vi "AB_RW_Project_Source_VI.vi"(7 "action":T3, 8 "error in (no error)":errorcluster, 9 "index in":i32, 10 "dataSource in":T2, 11 "buildObject":T1) -> (0 "error out":errorcluster, 1 "index out":i32, 2 "dataSource out":T2, 3 "buildObject out":T1)   [LabVIEW 2020]
doc: "Reads and writes the data to the object property bag."
uses:
  <resource>/Framework/Providers/API/ItemRef.ctl
  <vilib>/AppBuilder/RW_Project/AB_RW_Project_Source_VI_Data.ctl
  <vilib>/AppBuilder/RW_Project/AB_RW_Project_PropBag_Action.ctl
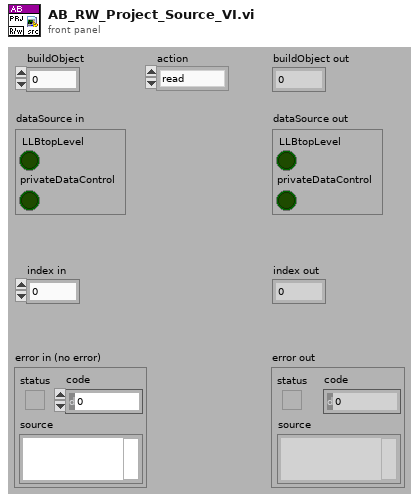
[diagram p1: front panel]
types:
  T1 = typedef "ItemRef.ctl" = u64
  T2 = typedef "AB_RW_Project_Source_VI_Data.ctl" = cluster{"LLBtopLevel":bool, "privateDataControl":bool}
  T3 = typedef "AB_RW_Project_PropBag_Action.ctl" = enum16{"read", "write", "clear", "readPrevious", "writePrevious", "clearPrevious"}
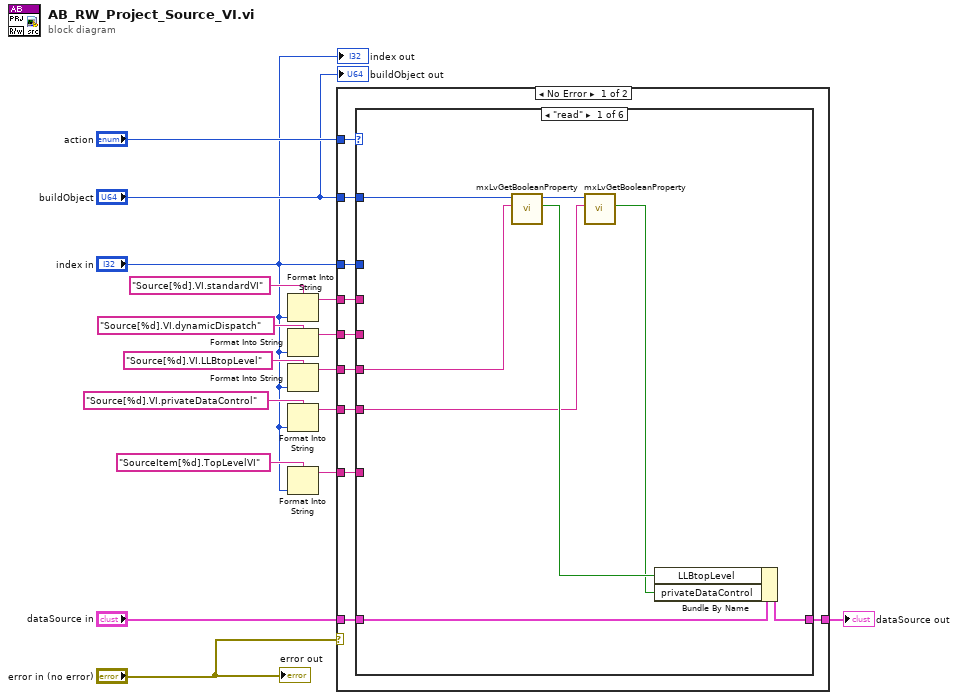
[diagram p0: block diagram]
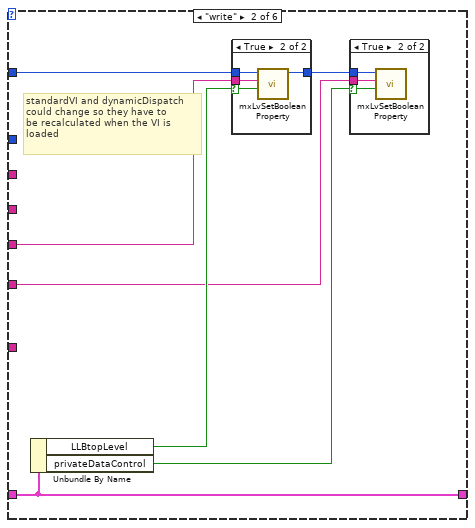
[diagram p2: hidden frame]
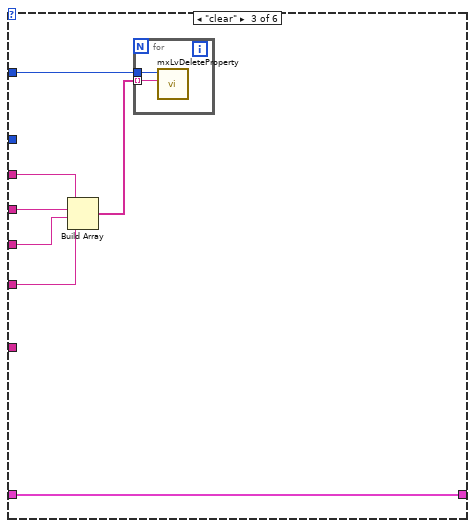
[diagram p5: hidden frame]
diagram:
  n1 = Format Into String(format string="Source[%d].VI.standardVI", "index in") -> (resulting string=w13:string)  [unwired: 2 in, 1 out]
  n2 = Format Into String(format string="Source[%d].VI.dynamicDispatch", "index in") -> (resulting string=w10:string)  [unwired: 2 in, 1 out]
  n3 = Format Into String(format string="Source[%d].VI.LLBtopLevel", "index in") -> (resulting string=w9:string)  [unwired: 2 in, 1 out]
  n4 = Format Into String(format string="Source[%d].VI.privateDataControl", "index in") -> (resulting string=w1:string)  [unwired: 2 in, 1 out]
  n5 = Format Into String(format string="SourceItem[%d].TopLevelVI", "index in") -> (resulting string=w4:string)  [unwired: 2 in, 1 out]
  n6 = case shown="No Error" "error in (no error)" {
    tunnel: "action" -> [w26 _]
    tunnel: "dataSource in" -> [w25 w62]
    tunnel: w13 -> [w24 _]
    tunnel: w10 -> [w23 _]
    tunnel: w9 -> [w22 _]
    tunnel: "index in" -> [w21 _]
    tunnel: [w20 w62] -> w8
    tunnel: "buildObject" -> [w19 _]
    tunnel: w4 -> [w18 _]
    tunnel: w1 -> [w17 _]
    frame No Error {
      n7 = case shown="\"read\"" w26 {
        tunnel: w19 -> [w30 w40 w51 _ _ _]
        tunnel: w25 -> [w34 w41 w56 w59 w60 w61]
        tunnel: w24 -> [_ _ w55 _ _ _]
        tunnel: w23 -> [_ _ w54 _ _ _]
        tunnel: w22 -> [w32 w39 w53 _ _ _]
        tunnel: w21 -> [_ _ _ _ _ _]
        tunnel: [w33 w41 w56 w59 w60 w61] -> w20
        tunnel: w18 -> [_ _ _ _ _ _]
        tunnel: w17 -> [w29 w36 w50 _ _ _]
        frame "read" {
          n8 = call <resource>:"mxLvGetBooleanProperty.vi"("Tag"=w32, "Item"=w30) -> ("Value"=w31:bool, "Item"=w28:T1)  [unwired: 7 in, 1 out]
          n9 = call <resource>:"mxLvGetBooleanProperty.vi"("Tag"=w29, "Item"=w28) -> ("Value"=w27:bool)  [unwired: 7 in, 2 out]
          n10 = Bundle By Name(cluster=w34, "LLBtopLevel"=w31, "privateDataControl"=w27) -> (w33:T2)
        }
        frame "write" {
          # "standardVI and dynamicDispatch\ncould change so they have to\nbe recalculated when the VI is\nloaded"
          n11 = Unbundle By Name(w41) -> ("LLBtopLevel"=w38:bool, "privateDataControl"=w35:bool)
          n12 = case shown="True" w38 {
            selector: w38 -> [_ w47]
            tunnel: w40 -> [w45 w49]
            tunnel: w39 -> [_ w48]
            tunnel: [w45 w46] -> w37
            frame False {
            }
            frame True {
              n13 = call <resource>:"mxLvSetBooleanProperty.vi"("Value (F)"=w47, "Tag"=w48, "Item"=w49) -> ("Item"=w46:T1)  [unwired: 7 in, 1 out]
            }
          }
          n14 = case shown="True" w35 {
            selector: w35 -> [_ w42]
            tunnel: w37 -> [_ w44]
            tunnel: w36 -> [_ w43]
            frame False {
            }
            frame True {
              n15 = call <resource>:"mxLvSetBooleanProperty.vi"("Value (F)"=w42, "Tag"=w43, "Item"=w44) -> ()  [unwired: 7 in, 2 out]
            }
          }
        }
        frame "clear" {
          n16 = Build Array(w55, w54, w53, w50) -> (w52:string[])
          n17 = for {
            tunnel: w51 -> [w58]
            tunnel: w52 -> [w57] mode=indexing
            n18 = call <resource>:"mxLvDeleteProperty.vi"("Tag"=w57, "Item"=w58) -> ()  [unwired: 8 in, 2 out]
          }
        }
        frame "readPrevious" {
        }
        frame "writePrevious" {
        }
        frame "clearPrevious" {
        }
      }
    }
    frame Error {
    }
  }
  "dataSource out" <- w8
  "error out" <- "error in (no error)"
  "buildObject out" <- "buildObject"
  "index out" <- "index in"
